vi "index power set-get all subsets.vi"(8 "error in (no error)":errorcluster, 11 "End index":i32=5) -> (0 "error out":errorcluster, 1 "Execution time (ms)":u32, 2 "no. of subsets":i32, 3 "Subsets of indexes":variant[](array[variant]))   [LabVIEW 2021, in "Numeric Utilities.lvlib"]
uses:
  Numeric Utilities.lvlib
  Named Timers/Named Timers.lvlib
panel:
  in  "Dev: Stop Button":bool
  # "Development\ncontrols/indicators useful for development and testing, but which are not outputs of the VI"
  # "Input\nInputs to the VI"
  # "Output\nOutputs of the VI"
  # "Description\n\nBlank VI with error handling case. \n\nSummarize the use of this VI in this space."
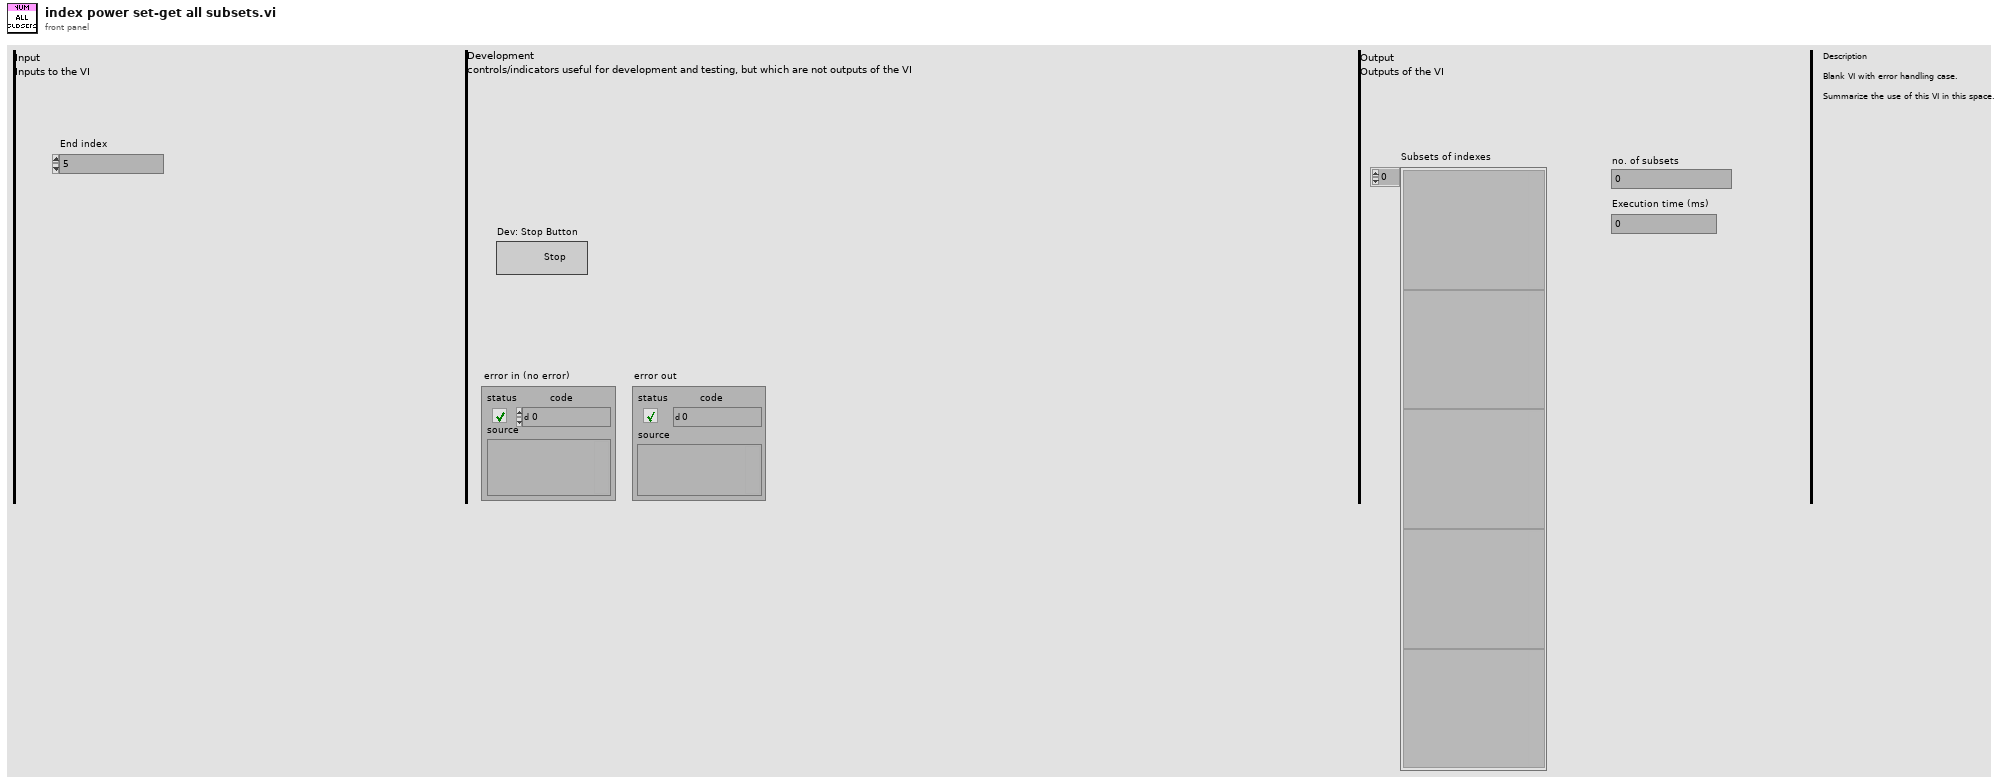
[diagram p1: front panel]
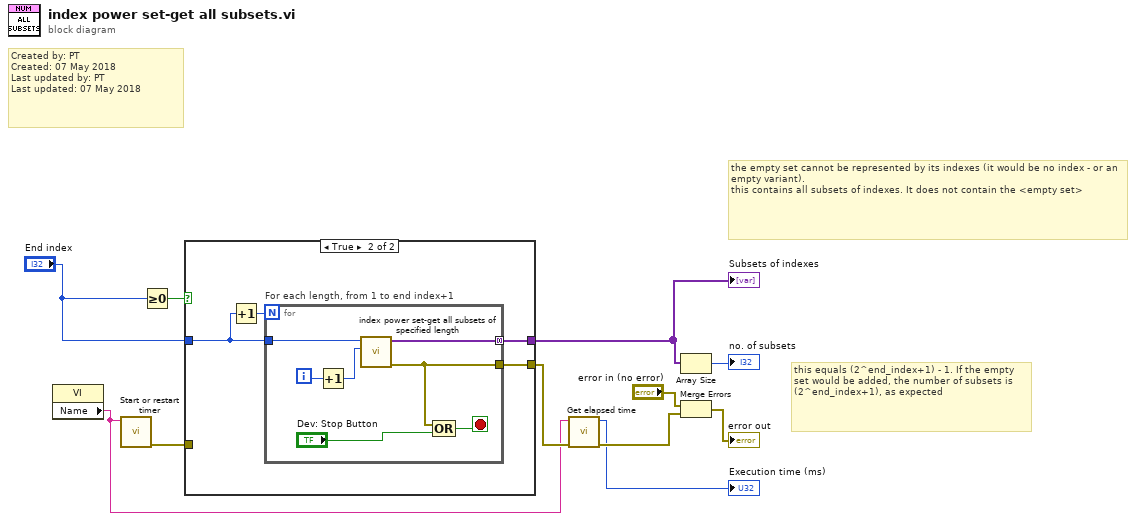
[diagram p0: block diagram]
diagram:
  # "this equals (2^end_index+1) - 1. If the empty set would be added, the number of subsets is (2^end_index+1), as expected"
  # "the empty set cannot be represented by its indexes (it would be no index - or an empty variant).\nthis contains all subsets of indexes. It does not contain the <empty set>"
  # "Created by: PT\nCreated: 07 May 2018\nLast updated by: PT\nLast updated: 07 May 2018"
  n1 = property class="VI"() -> ("Name"=w1:string)  [unwired: 2 in, 2 out]
  n2 = call "Start or restart timer.vi"("Timer name"=w1) -> ("error out"=w4:errorcluster)  [unwired: 10 in]
  n3 = Greater Or Equal To 0?(x="End index") -> (x >= 0?=w8:bool)
  n4 = case shown="True" w8 {
    tunnel: "End index" -> [_ w15]
    tunnel: [_ w13] -> w5
    tunnel: [_ w12] -> w6
    tunnel: w4 -> [_ _]
    frame False {
    }
    frame True {
      n5 = Increment(x=w15) -> (x+1=w14:i32)
      n6 = for "For each length, from 1 to end index+1" {
        N: w14 -> [_]
        tunnel: w15 -> [w22]
        tunnel: [w19] -> w13 mode=concatenating
        tunnel: [w18] -> w12
        i -> [w21]
        stop <- w17 stop-if-true
        n7 = Increment(x=w21) -> (x+1=w20:i32)
        n8 = call "index power set-get all subsets of specified length.vi"("Desired subsets length"=w20, "End index"=w22) -> ("error out"=w18:errorcluster, "Subsets of indexes"=w19:variant[])  [unwired: 7 in, 1 out]
        n9 = Compound Arithmetic op=OR(w18, "Dev: Stop Button") -> (w17:bool)
      }
    }
  }
  "Subsets of indexes" <- w5
  n10 = call "Get elapsed time.vi"("error in (no error)"=w6, "Timer name"=w1) -> ("error out"=w3:errorcluster, "Elapsed time (ms)"=→"Execution time (ms)":u32)  [unwired: 6 in, 2 out]
  n11 = Array Size(array=w5) -> (size(s)=→"no. of subsets":i32)
  n12 = Merge Errors("error in (no error)", w3) -> (→"error out":errorcluster)
